vi "Anritsu VNA Set Number of Points.vi"(6 "Channel":i8=1 min=1 step=1, 7 "Anritsu VNA":T1, 8 "error in (no error)":errorcluster, 10 "Number Points":i32, 11 "VISA Resource Name":refnum<visa-resource-name>) -> (0 "error out":errorcluster, 3 "dup VISA Resource Name":refnum<visa-resource-name>)   [LabVIEW 2011]
doc: "This VI for the HP 8753B is used to read the number of stimulus points."
uses:
  TypeDefs/Anritsu VNA Instrument Info.ctl
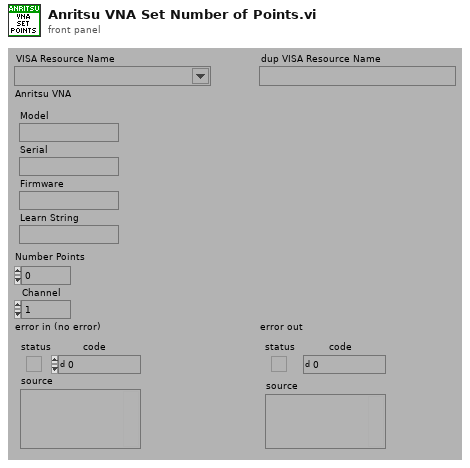
[diagram p1: front panel]
types:
  T1 = typedef "Anritsu VNA Instrument Info.ctl" = cluster{"Model":string, "Serial":string, "Firmware":string, "Learn String":string}
  T2 = typedef "Anritsu VNA Model.ctl" = enum16{"Not Supported", "37XXXX", "MS20XXX", "MS462XX", "MS464XX"}
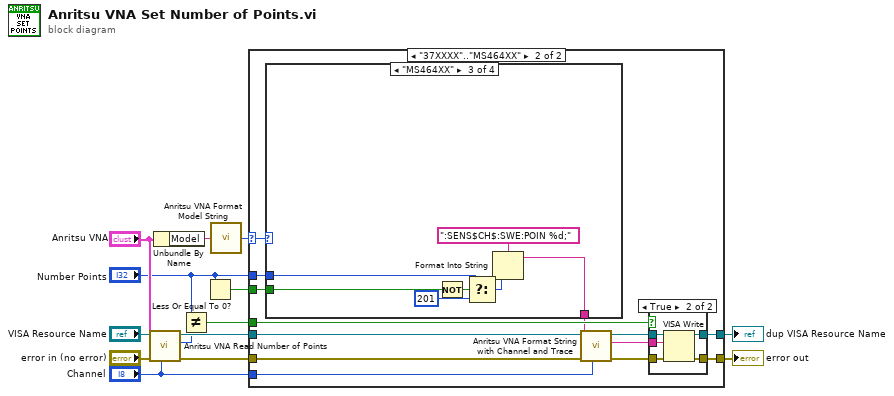
[diagram p0: block diagram]
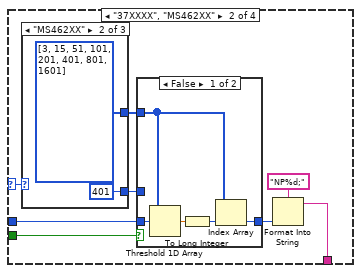
[diagram p4: hidden frame]
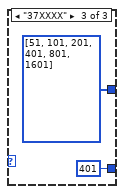
[diagram p6: hidden frame]
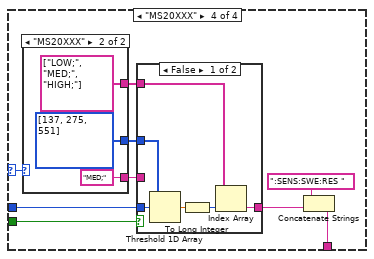
[diagram p8: hidden frame]
diagram:
  n1 = call "Anritsu VNA Read Number of Points.vi"("Channel"="Channel", "Anritsu VNA"="Anritsu VNA", "error in (no error)"="error in (no error)", "VISA Resource Name"="VISA Resource Name") -> ("error out"=w8:errorcluster, "Number Points"=w7:i32, "dup VISA Resource Name"=w9:refnum<visa-resource-name>)  [unwired: 5 out]
  n2 = Unbundle By Name("Anritsu VNA") -> ("Model"=w3:string)
  n3 = Not Equal?(x="Number Points", y=w7) -> (x != y?=w12:bool)
  n4 = Less Or Equal To 0?(x="Number Points") -> (x <= 0?=w4:bool)
  n5 = call "Anritsu VNA Format Model String.vi"("Model"=w3) -> ("Model"=w2:T2)
  n6 = case shown="\"37XXXX\"..\"MS464XX\"" w2 {
    selector: w2 -> [_ w20]
    tunnel: [w16 w27] -> w14
    tunnel: [w15 w26] -> w13
    tunnel: w12 -> [_ w25]
    tunnel: w9 -> [w16 w24]
    tunnel: w8 -> [w15 w23]
    tunnel: "Number Points" -> [_ w22]
    tunnel: w4 -> [_ w21]
    tunnel: "Channel" -> [_ w17]
    frame "Not Supported" {
    }
    frame "37XXXX".."MS464XX" {
      n7 = case shown="\"MS464XX\"" w20 {
        selector: w20 -> [_ w28 _ w54]
        tunnel: [_ w29 w51 w61] -> w19
        tunnel: w22 -> [_ w33 w47 w60]
        tunnel: w21 -> [_ w32 w50 w53]
        frame "Not Supported" {
        }
        frame "37XXXX", "MS462XX" {
          n8 = case shown="\"MS462XX\"" w28 {
            tunnel: [_ 401 401] -> w34
            tunnel: [_ i32[] [3, 15, 51, 101, 201, 401, 801, 1601] i32[] [51, 101, 201, 401, 801, 1601]] -> w35
            frame "Not Supported", "MS20XXX", "MS464XX" {
            }
            frame "MS462XX" {
            }
            frame "37XXXX" {
            }
          }
          n9 = case shown="False" w32 {
            tunnel: [w42 w45] -> w31
            tunnel: w33 -> [w41 _]
            tunnel: w34 -> [_ w45]
            tunnel: w35 -> [w40 _]
            frame False {
              n10 = Threshold 1D Array(2:w41, 3:w40) -> (0:w44:dbl)  [unwired: 1 out]
              n11 = To Long Integer(number=w44) -> (32bit integer=w43:i32)
              n12 = Index Array(array=w40, index=w43) -> (element=w42:i32)
            }
            frame True {
            }
          }
          n13 = Format Into String(format string="NP%d;", w31) -> (resulting string=w29:string)  [unwired: 2 in, 1 out]
        }
        frame "MS464XX" {
          n14 = Not(x=w50) -> (.not. x?=w49:bool)
          n15 = Select(t=w47, s=w49, f=201) -> (s? t:f=w46:i32)
          n16 = Format Into String(format string=":SENS$CH$:SWE:POIN %d;", w46) -> (resulting string=w51:string)  [unwired: 2 in, 1 out]
        }
        frame "MS20XXX" {
          n17 = case shown="\"MS20XXX\"" w54 {
            tunnel: [_ i32[] [137, 275, 551]] -> w59
            tunnel: [_ "MED;"] -> w58
            tunnel: [_ string[] ["LOW;", "MED;", "HIGH;"]] -> w57
            frame "Not Supported", "37XXXX", "MS462XX", "MS464XX" {
            }
            frame "MS20XXX" {
            }
          }
          n18 = case shown="False" w53 {
            tunnel: w59 -> [w66 _]
            tunnel: [w64 w68] -> w56
            tunnel: w60 -> [w63 _]
            tunnel: w58 -> [_ w68]
            tunnel: w57 -> [w62 _]
            frame False {
              n19 = Threshold 1D Array(2:w63, 3:w66) -> (0:w67:dbl)  [unwired: 1 out]
              n20 = To Long Integer(number=w67) -> (32bit integer=w65:i32)
              n21 = Index Array(array=w62, index=w65) -> (element=w64:string)
            }
            frame True {
            }
          }
          n22 = Concatenate Strings(":SENS:SWE:RES ", w56) -> (w61:string)
        }
      }
      n23 = call "Anritsu VNA Format String with Channel and Trace.vi"("Channel"=w17, "String"=w19) -> ("String Out"=w18:string)  [unwired: 1 in, 6 out]
      n24 = case shown="True" w25 {
        tunnel: w24 -> [w73 w78]
        tunnel: w23 -> [w72 w77]
        tunnel: [w73 w76] -> w27
        tunnel: [w72 w75] -> w26
        tunnel: w18 -> [_ w74]
        frame False {
        }
        frame True {
          n25 = VISA Write(VISA resource name=w78, write buffer=w74, error in (no error)=w77) -> (VISA resource name out=w76:refnum<visa-resource-name>, error out=w75:errorcluster)  [unwired: 1 out]
        }
      }
    }
  }
  "dup VISA Resource Name" <- w14
  "error out" <- w13
